vi "Adv_GetData.vi"(8 "error in (no error)":errorcluster, 10 "IImageDataSet":refnum<k24>, 11 "LightField Automation in":refnum<class "LightField Automation.lvclass">) -> (0 "error out":errorcluster, 2 "Data":T1(array[cluster]), 3 "LightField Automation out":refnum<class "LightField Automation.lvclass">)   [LabVIEW 2013, in "LightField Automation.lvclass"]
uses:
  LightField Automation.lvclass
  C:/Program Files/Princeton Instruments/LightField/AddInViews/PrincetonInstruments.LightFieldViewV3.dll
  Program Files/Princeton Instruments/LightField/AddInViews/PrincetonInstruments.LightFieldViewV3.dll
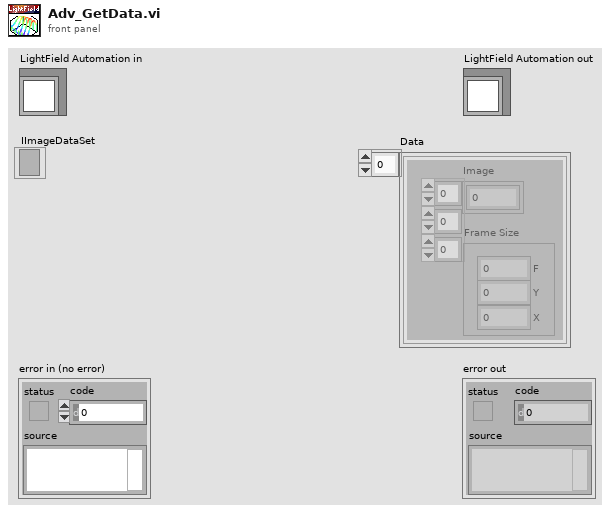
[diagram p1: front panel]
types:
  T1 = cluster{"Image":dbl[][][], "Frame Size":cluster{"F":i32, "Y":i32, "X":i32}}[]
  T2 = cluster{"Image":dbl[][][], "Frame Size":cluster{"F":i32, "Y":i32, "X":i32}}
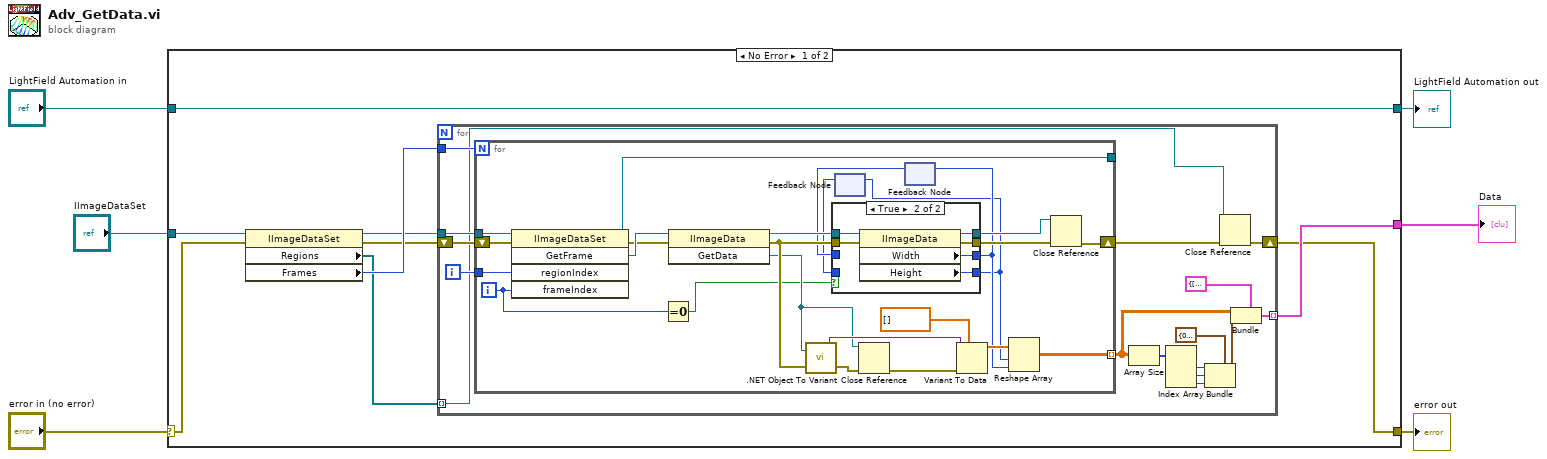
[diagram p0: block diagram]
diagram:
  n1 = case shown="No Error" "error in (no error)" {
    selector: "error in (no error)" -> [w9 w67]
    tunnel: [w7 w67] -> w5
    tunnel: [w8 w66] -> w3
    tunnel: "LightField Automation in" -> [w8 w66]
    tunnel: [w15 _] -> w2
    tunnel: "IImageDataSet" -> [w10 _]
    frame No Error {
      n2 = property class="IImageDataSet"(reference=w10, error in=w9) -> (reference out=w12:refnum<k24>, error out=w13:errorcluster, "Regions"=w11:refnum<k24>[], "Frames"=w14:i64)
      n3 = for {
        tunnel: w12 -> [w31]
        shift-right: [w17] -> w7
        shift-left: w13 -> [w30]
        tunnel: w14 -> [w29]
        tunnel: [w25] -> w15 mode=indexing
        tunnel: w11 -> [w16] mode=indexing
        i -> [w28]
        n4 = for {
          N: w29 -> [_]
          tunnel: w31 -> [w45]
          tunnel: w28 -> [w54]
          shift-right: [w42] -> w18
          shift-left: w30 -> [w55]
          tunnel: [w46] -> w26 mode=indexing
          tunnel: [w41] -> _
          i -> [w37]
          n5 = invoke class="IImageDataSet" method="GetFrame"(reference=w45, error in=w55, "regionIndex"=w54, "frameIndex"=w37) -> (reference out=w41:refnum<k24>, error out=w52:errorcluster, "GetFrame"=w53:refnum<k24>)  [unwired: 1 in, 2 out]
          n6 = Equal To 0?(x=w37) -> (x = 0?=w36:bool)
          n7 = invoke class="IImageData" method="GetData"(reference=w53, error in=w52) -> (reference out=w51:refnum<k24>, error out=w50:errorcluster, "GetData"=w38:refnum<k24>)  [unwired: 1 in]
          n8 = call <vilib>:".NET Object To Variant.vi"("error in (no error)"=w50, ".NET object"=w38) -> ("error out"=w39:errorcluster, "variant"=w49:variant)
          n9 = feedback #1() -> (w32:i32)  [unwired: 1 in]
          n10 = Close Reference(reference=w38, error in (no error)=w39) -> (error out=w40:errorcluster)
          n11 = feedback #2() -> (w33:i32)  [unwired: 1 in]
          n12 = case shown="True" w36 {
            tunnel: w51 -> [w59 w65]
            tunnel: w50 -> [w58 w64]
            tunnel: [w57 w63] -> w35
            tunnel: [w56 w62] -> w34
            tunnel: [w58 w61] -> w44
            tunnel: [w59 w60] -> w43
            tunnel: w33 -> [w57 _]
            tunnel: w32 -> [w56 _]
            frame False {
            }
            frame True {
              n13 = property class="IImageData"(reference=w65, error in=w64) -> (reference out=w60:refnum<k24>, error out=w61:errorcluster, "Width"=w63:i32, "Height"=w62:i32)
            }
          }
          n14 = feedback-in #1(w34) -> ()
          n15 = feedback-in #2(w35) -> ()
          n16 = Variant To Data(error in=w40, type=dbl[] [], Variant=w49) -> (data=w47:dbl[])  [unwired: 1 out]
          n17 = Reshape Array(w47, w34, w35) -> (w46:dbl[][])
          n18 = Close Reference(reference=w43, error in (no error)=w44) -> (error out=w42:errorcluster)
        }
        n19 = Array Size(array=w26) -> (size(s)=w27:i32[])
        n20 = Index Array(array=w27) -> (element #1=w23:i32, element #2=w24:i32, element #3=w22:i32)  [unwired: 3 in]
        n21 = Bundle(cluster=cluster{"F":i32, "Y":i32, "X":i32} {"F"=0, "Y"=0, "X"=0} ("Frame Size"), "F"=w23, "Y"=w24, "X"=w22) -> (w19:cluster{"F":i32, "Y":i32, "X":i32})
        n22 = Close Reference(reference=w16, error in (no error)=w18) -> (error out=w17:errorcluster)
        n23 = Bundle(cluster=T2 {"Image"=[], "Frame Size"={"F"=0, "Y"=0, "X"=0}} ("Cluster"), "Image"=w26, "Frame Size"=w19) -> (w25:T2)
      }
    }
    frame Error {
    }
  }
  "error out" <- w5
  "LightField Automation out" <- w3
  "Data" <- w2
